vi "Register Dynamic Status Change Event.vi"() -> ()   [LabVIEW 2014]
uses:
  user.lib/_NEVSTOP/JKI State Machine ++/_Support/_JKISMQFGV.vi
  user.lib/_NEVSTOP/JKI State Machine ++/_Support/FGV-BroadcastRegistry/FGV-BroadcastRegistry.vi
  user.lib/_NEVSTOP/JKI State Machine ++/JKI-State-Machine-Plus.lvlib
panel:
  in  "unRegister":bool
  in  "Register":bool
  out "State History 2":string
  in  "Start SubModule":bool
  out "State History":string
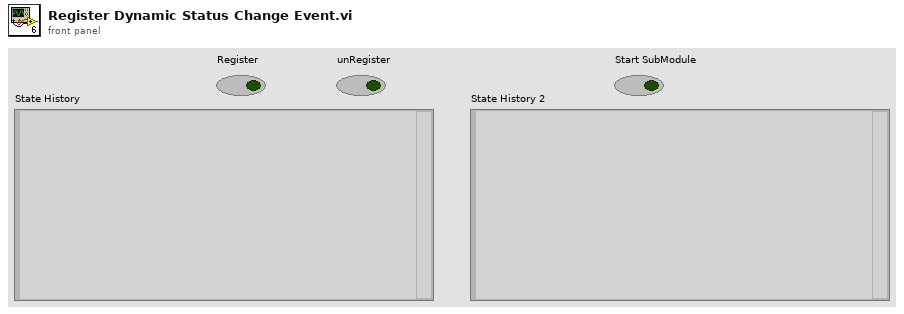
[diagram p1: front panel]
types:
  T1 = enum32{"Invalid", "Standard", "Closed", "Hidden", "Minimized", "Maximized"}
  T2 = enum32{"invalid app kind", "Development System", "Run Time System", "Student Edition", "Embedded LabVIEW", "Evaluation", "Custom"}
  T3 = cluster{"Core":cluster{"Current VI Reference":refnum<vi>, "Close Panel on Exit?":bool}, "Your Boolean data":bool, "Your string data":string}
  T4 = cluster{"Current VI Reference":refnum<vi>, "Close Panel on Exit?":bool}
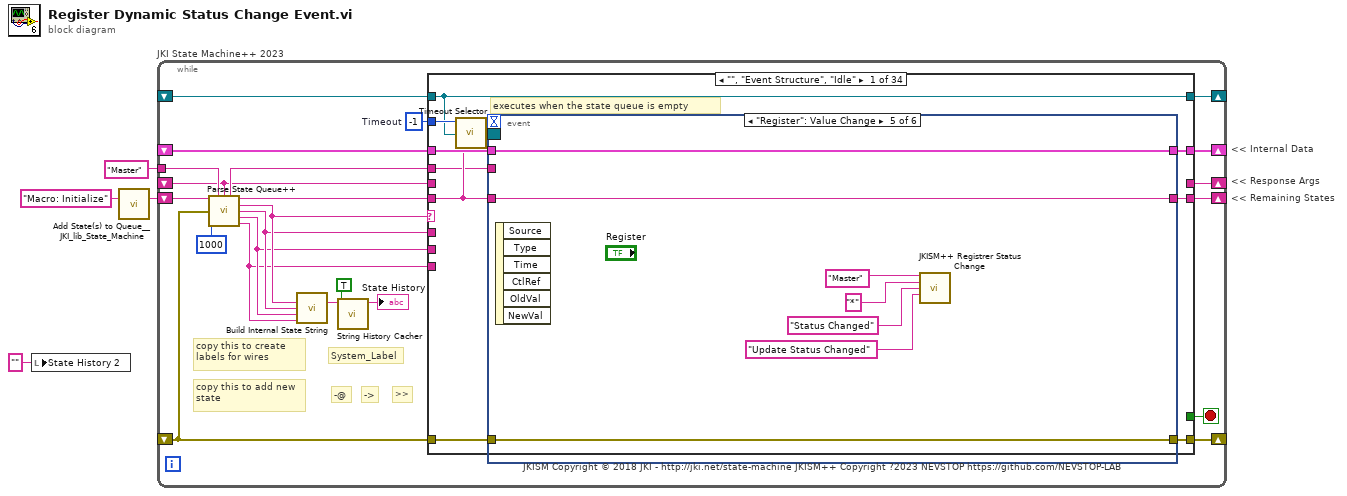
[diagram p0: block diagram]
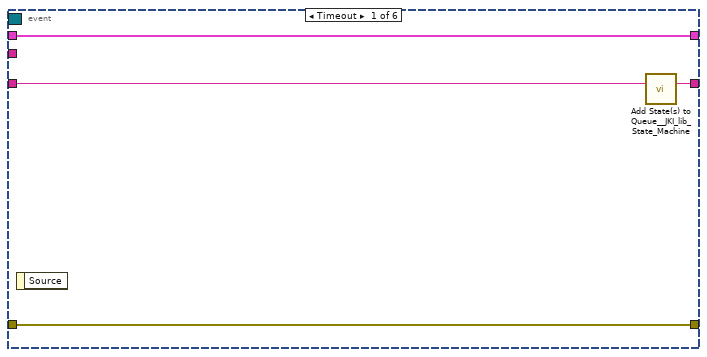
[diagram p2: hidden frame]
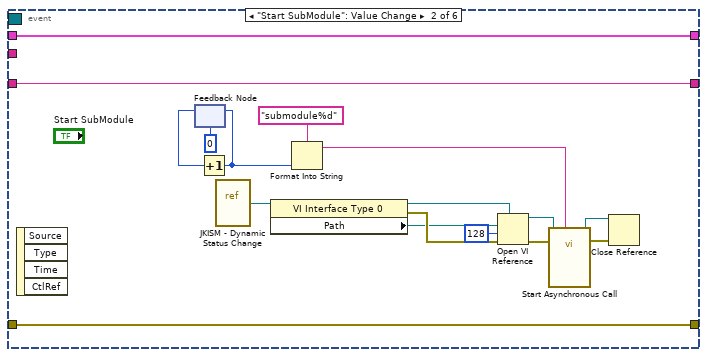
[diagram p3: hidden frame]
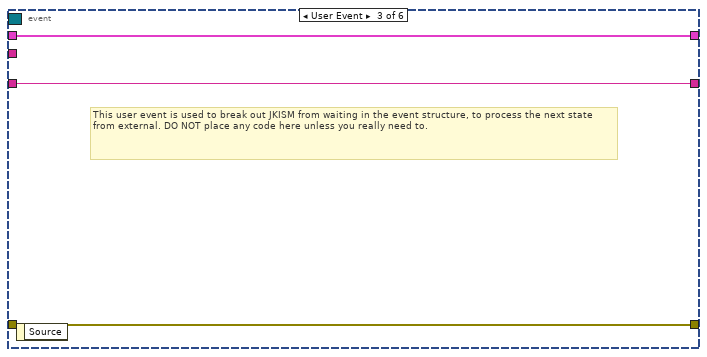
[diagram p4: hidden frame]
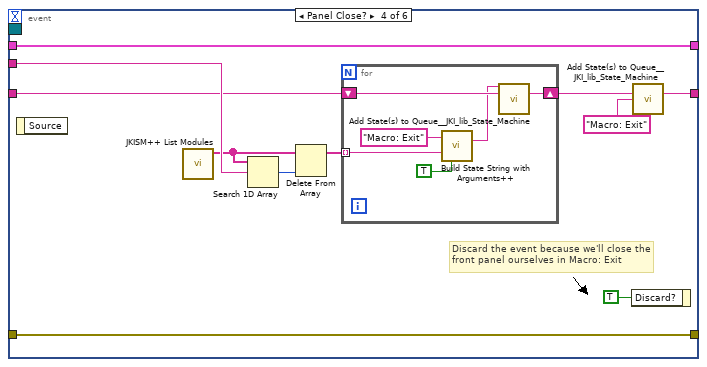
[diagram p5: hidden frame]
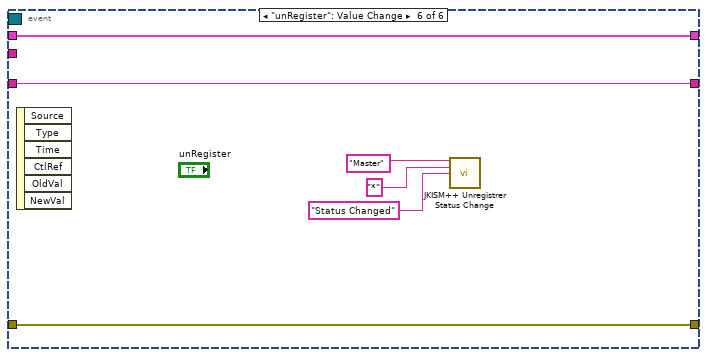
[diagram p6: hidden frame]
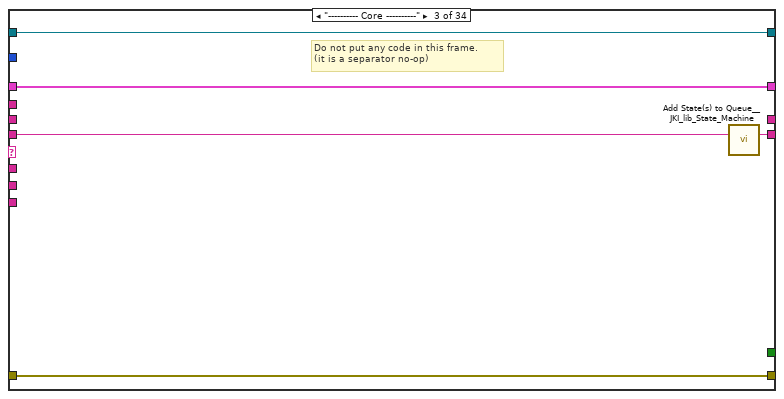
[diagram p8: hidden frame]
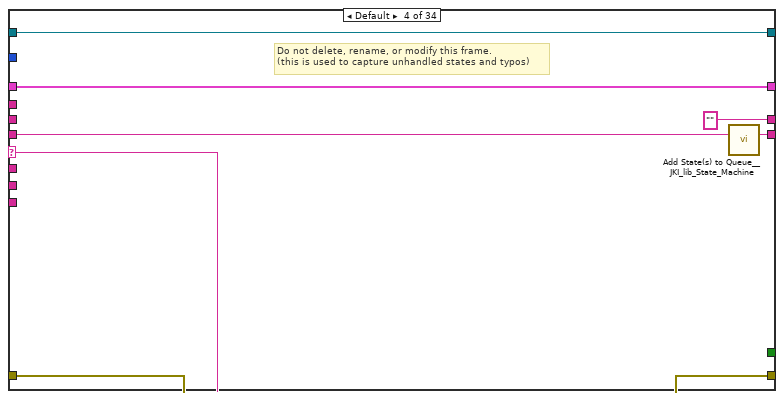
[diagram p9: hidden frame]
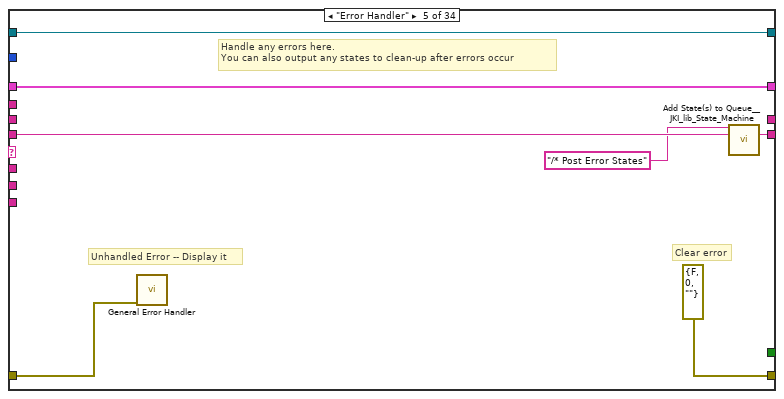
[diagram p10: hidden frame]
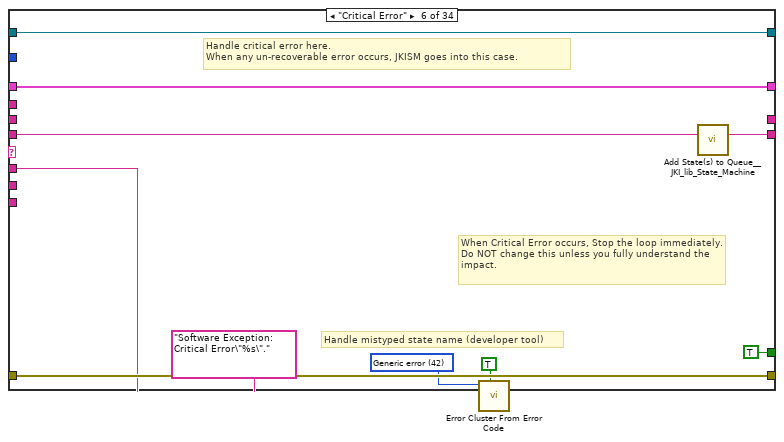
[diagram p11: hidden frame]
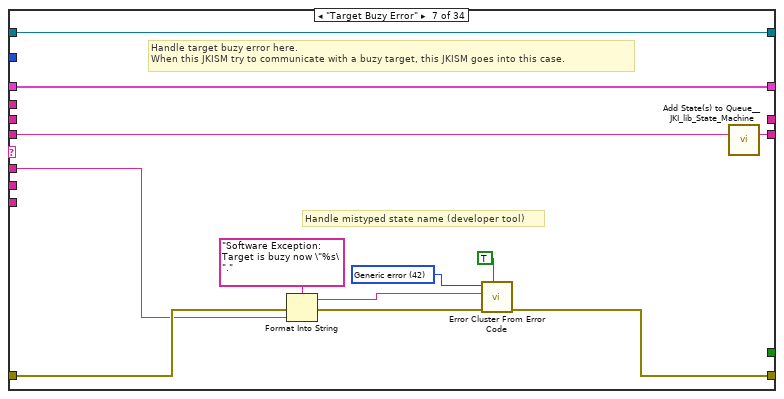
[diagram p12: hidden frame]
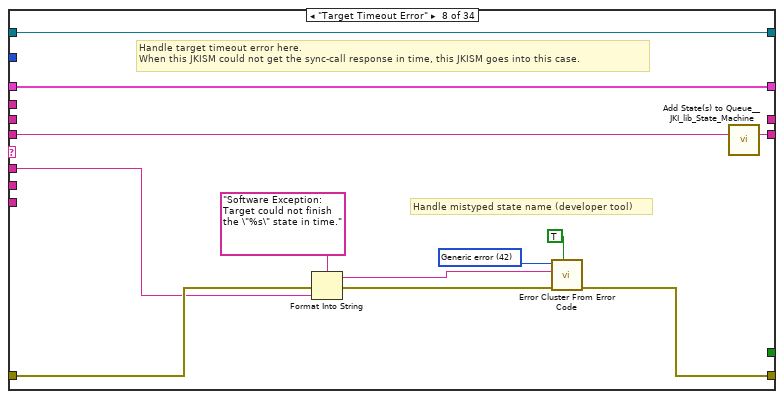
[diagram p13: hidden frame]
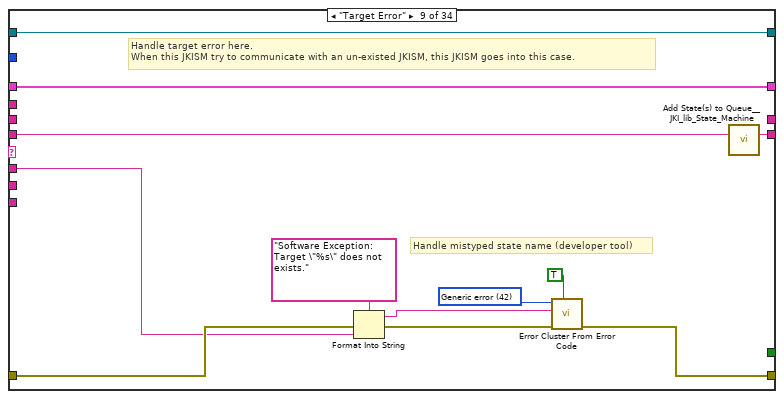
[diagram p14: hidden frame]
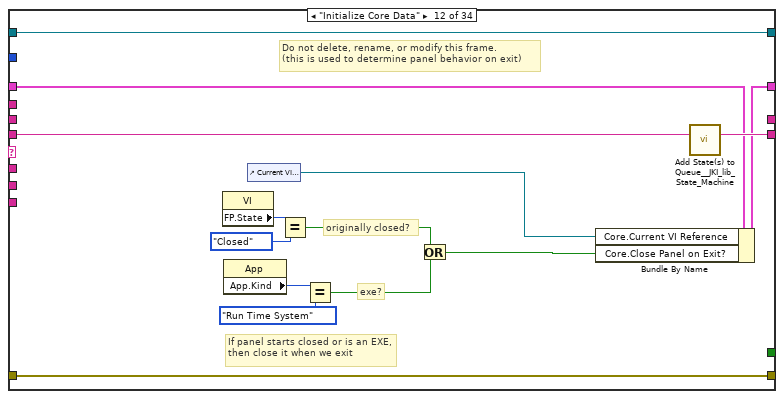
[diagram p17: hidden frame]
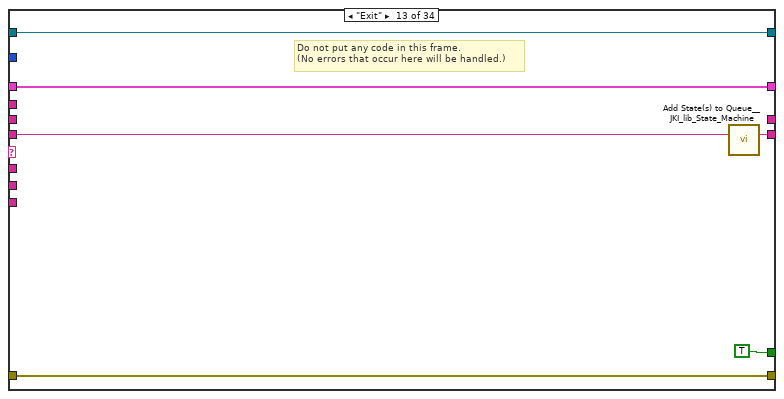
[diagram p18: hidden frame]
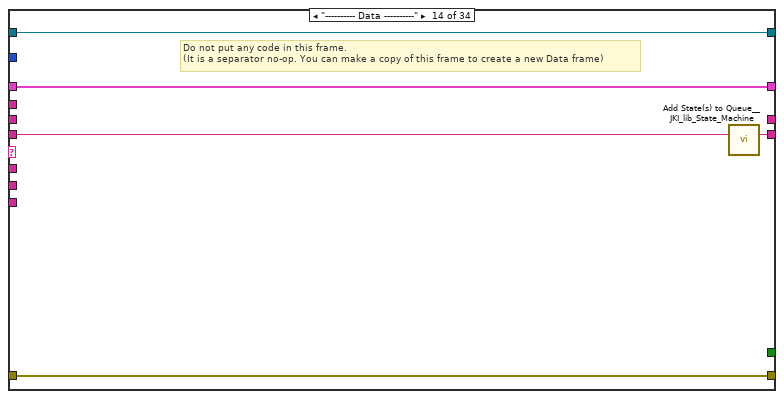
[diagram p19: hidden frame]
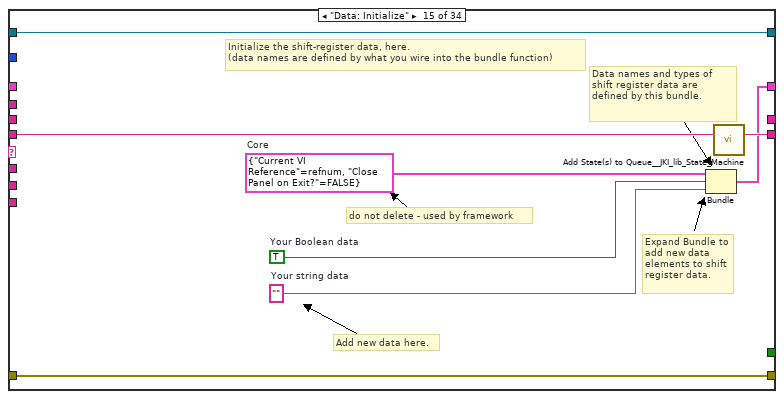
[diagram p20: hidden frame]
diagram:
  # "<< Internal Data"
  # "<< Response Args"
  # "<< Remaining States"
  n1 = local write "State History 2"("" ("State History 2")) -> ()
  n2 = call <vilib>:"Add State(s) to Queue__JKI_lib_State_Machine.vi"("State(s) in (\"\")"="Macro: Initialize") -> ("States Out"=w4:string)  [unwired: 14 in]
  n3 = while "JKI State Machine++ 2023" {
    shift-right: [w22] -> _
    shift-left: _ -> [w21]
    shift-right: [w25] -> _
    shift-left: _ -> [w19]
    shift-right: [w24] -> _
    shift-left: w4 -> [w26]
    tunnel: "Master" ("Name(\"\" to use uuid)") -> [w14]
    shift-right: [w17] -> _
    shift-left: _ -> [w6]
    shift-right: [w16] -> _
    shift-left: _ -> [w15]
    stop <- w23 stop-if-true
    w20 = -1  # Timeout
    # "JKISM Copyright © 2018 JKI - http://jki.net/state-machine JKISM++ Copyright ?2023 NEVSTOP https://github.com/NEVSTOP-LAB"
    # "copy this to add new state"
    # ">>"
    # "->"
    # "-@"
    # "copy this to create labels for wires"
    # "System_Label"
    n4 = call "Parse State Queue++.vi"("State Queue"=w26, "Name(\"\" to use uuid)"=w14, "Response Arguments"=w6, "Error In (no error)"=w19, "Response Timeout(5000ms)"=1000 ("Response Timeout(1000ms)")) -> ("Name Used"=w7:string, "Remaining States"=w27:string, "Current State"=w11:string, "Arguments"=w10:string, "Argument - State"=w9:string, "From Who"=w8:string)  [unwired: 5 in]
    n5 = call "Build Internal State String.vi"("State"=w11, "Arguments (\"\")"=w10, "Arg-State (\"\")"=w9, "Source (\"\")"=w8) -> ("State with Arguments"=w12:string)  [unwired: 11 in]
    n6 = call "String History Cacher.vi"("Include Timestamp(F)"=TRUE, "String"=w12) -> ("String Cache"=→"State History":string)  [unwired: 9 in]
    n7 = case shown="\"\", \"Event Structure\", \"Idle\"" w11 {
      selector: w11 -> [_ _ _ w103 _ _ _ _ _ _ _ _ _ _ _ _ _ _ _ _ _ _ _ _ _ _ _ _ _ _ _ _ _ _]
      tunnel: w27 -> [w29 w94 w100 w107 w120 w130 w133 w150 w162 w171 w175 w190 w196 w201 w209 w216 w221 w227 w231 w237 w242 w249 w261 w331 w337 w348 w351 w356 w362 w370 w376 w384 w391 w405]
      tunnel: w10 -> [_ _ _ _ _ w123 w135 w146 w158 _ _ _ _ _ _ _ _ _ _ _ _ w244 w255 _ _ _ _ _ w359 _ _ w378 _ w402]
      tunnel: w21 -> [w36 w93 w97 w105 w117 w131 w137 w148 w160 w170 w174 w183 w194 w198 _ w211 w218 w226 w230 w234 w240 w247 w257 w328 w334 w345 w350 w355 w361 w367 w373 w383 w388 w404]
      tunnel: [w35 w95 w98 w109 errorcluster {"status"=FALSE, "code"=0, "source"=""} ("error out") w132 w140 w152 w164 w172 w176 w187 w193 w199 w206 w212 w219 w222 w229 w235 w239 w245 w258 w329 w335 w346 w352 w357 w363 w368 w374 w385 w389 w406] -> w25
      tunnel: w19 -> [w34 w95 w98 w108 w116 w132 w139 w151 w163 w172 w176 w187 w193 w199 w206 w213 w219 _ w232 w235 w239 w246 w259 w329 w335 w346 w352 w357 w363 w368 w374 w385 w389 w406]
      tunnel: [w37 w94 w99 w106 w119 w129 w138 w149 w161 w171 w175 w189 w195 w200 w208 w215 w220 w227 w231 w236 w241 w248 w260 w330 w336 w347 w351 w356 w362 w369 w375 w384 w390 w405] -> w24
      tunnel: [_ _ _ _ _ TRUE _ _ _ _ _ _ TRUE _ _ _ _ _ _ _ _ _ _ _ _ _ _ _ _ _ _ _ _ _] -> w23
      tunnel: [w33 w93 w97 w105 w117 w131 w137 w148 w160 w170 w174 w188 w194 w198 w207 w211 w218 w226 w230 w234 w240 w247 w257 w328 w334 w345 w350 w355 w361 w367 w373 w383 w388 w404] -> w22
      tunnel: w20 -> [w32 _ _ _ _ _ _ _ _ _ _ _ _ _ _ _ _ _ _ _ _ _ _ _ _ _ _ _ _ _ _ _ _ _]
      tunnel: w8 -> [_ _ _ _ _ _ _ _ _ _ _ _ _ _ _ _ _ _ _ _ _ _ _ _ _ _ _ _ _ _ _ w379 _ w397]
      tunnel: w9 -> [_ _ _ _ _ _ _ _ _ _ _ _ _ _ _ _ _ _ _ _ _ _ _ _ _ _ _ _ _ _ _ _ _ w396]
      tunnel: [_ _ _ "" _ _ _ _ _ _ _ _ _ _ _ _ _ _ _ _ _ _ _ _ _ _ _ "API1 Response" w358 _ "DoA Finished" _ "DoB Finished" _] -> w17
      tunnel: [w31 w92 w96 w101 w114 w121 w134 w145 w157 w169 w173 w177 w191 w197 w202 w210 w217 w225 w228 w233 w238 w243 w254 w327 w332 w338 w349 w354 w360 w366 w372 w382 w387 w403] -> w16
      tunnel: w15 -> [w31 w92 w96 w101 w114 w121 w134 w145 w157 w169 w173 w177 w191 w197 w202 w210 w217 _ w228 w233 w238 w243 w254 w327 w332 w338 w349 w354 w360 w366 w372 w382 w387 w403]
      tunnel: w7 -> [w28 _ _ _ _ _ _ _ _ _ _ _ _ _ _ _ _ w224 _ _ _ _ _ _ _ _ _ _ _ _ _ _ _ _]
      tunnel: w6 -> [_ _ _ _ _ _ _ _ _ _ _ _ _ _ _ _ _ _ _ _ _ _ _ _ _ _ _ _ _ _ _ _ _ _]
      frame "", "Event Structure", "Idle" {
        # "executes when the state queue is empty"
        n8 = call "Timeout Selector.vi"("Remaining States"=w29, "Timeout Expected"=w32) -> ("Timeout"=w30:i32)  [unwired: 5 in]
        n9 = event shown="[4] \"Register\": Value Change" {
          selector: w31 -> [_ _ _ _ _ _]
          dyn-events: _ -> [_ _ _ _ _ _]
          timeout: w30 -> [_ _ _ _ _ _]
          tunnel: w29 -> [w41 w58 w60 w63 w85 w91]
          tunnel: [w40 w58 w60 w72 w85 w91] -> w37
          tunnel: w36 -> [w38 w56 w61 w70 w83 w89]
          tunnel: [w39 w57 w59 w71 w84 w90] -> w35
          tunnel: w34 -> [w39 w57 w59 w71 w84 w90]
          tunnel: [w38 w56 w61 w70 w83 w89] -> w33
          tunnel: w28 -> [_ _ _ w68 _ _]
          event Timeout {
            n10 = event-data() -> ()  [unwired: 1 in, 1 out]
            n11 = call <vilib>:"Add State(s) to Queue__JKI_lib_State_Machine.vi"("State(s) in (\"\")"=w41) -> ("States Out"=w40:string)  [unwired: 14 in]
          }
          event "Start SubModule": Value Change {
            n12 = event-data() -> ()  [unwired: 1 in, 4 out]
            n13 = feedback #1(0 ("Response Timeout(1000ms)")) -> (w54:i32)
            n14 = Increment(x=w54) -> (x+1=w44:i32)
            n15 = feedback-in #1(w44) -> ()
            n16 = vi-ref "JKISM - Dynamic Status Change.vi"() -> (w46:refnum<vi>)
            n17 = property class="VI Interface Type 0"(reference=w46) -> (reference out=w50:refnum<vi>, error out=w48:errorcluster, "Path"=w47:path)  [unwired: 1 in]
            n18 = Format Into String(format string="submodule%d", w44) -> (resulting string=w42:string)  [unwired: 2 in, 1 out]
            n19 = Open VI Reference(type specifier VI Refnum (for type only)=w50, vi path=w47, options=128, error in (no error)=w48) -> (vi reference=w49:refnum<vi>, error out=w45:errorcluster)  [unwired: 2 in]
            n20 = call-by-ref "Start Asynchronous Call"(reference=w49, error in=w45, "Name(\"\" to use uuid)"=w42) -> (reference out=w52:refnum<vi>, error out=w51:errorcluster)  [unwired: 11 in]
            n21 = Close Reference(reference=w52, error in (no error)=w51) -> ()  [unwired: 1 out]
          }
          event User Event {
            # "This user event is used to break out JKISM from waiting in the event structure, to process the next state from external. DO NOT place any code here unless you really need to."
            n22 = event-data() -> ()  [unwired: 1 in, 1 out]
          }
          event Panel Close? {
            # "Discard the event because we'll close the front panel ourselves in Macro: Exit"
            n23 = event-data() -> ()  [unwired: 1 in, 1 out]
            n24 = call "JKISM++ List Modules.vi"() -> ("Name"=w67:string[])  [unwired: 10 in, 1 out]
            n25 = Search 1D Array(1D array=w67, element=w68) -> (index of element=w66:i32)  [unwired: 1 in]
            n26 = Delete From Array(array=w67, index=w66) -> (array with subset deleted=w65:string[])  [unwired: 1 in, 1 out]
            n27 = for {
              tunnel: w65 -> [w78] mode=indexing
              shift-right: [w75] -> w64
              shift-left: w63 -> [w74]
              n28 = call "Build State String with Arguments++.vi"("State"="Macro: Exit", "Dest Module (\"\")"=w78, "Sync-Call(@) T By Default/Async-Call(->) F"=TRUE) -> ("State with Arguments"=w73:string)  [unwired: 12 in]
              n29 = call <vilib>:"Add State(s) to Queue__JKI_lib_State_Machine.vi"("State(s) in Front (\"\")"=w73, "State(s) in (\"\")"=w74) -> ("States Out"=w75:string)  [unwired: 13 in]
            }
            n30 = event-data("Discard?"=TRUE) -> ()  [unwired: 1 in, 1 out]
            n31 = call <vilib>:"Add State(s) to Queue__JKI_lib_State_Machine.vi"("State(s) in (\"\")"=w64, "State(s) at Back (\"\")"="Macro: Exit") -> ("States Out"=w72:string)  [unwired: 13 in]
          }
          event "Register": Value Change {
            n32 = event-data() -> ()  [unwired: 1 in, 6 out]
            n33 = call "JKISM++ Registrer Status Change.vi"("JKISM Name"="Master" ("Source JKISM Name"), "Source JKISM Name (* as Default)"="*" ("Name(\"\" to use uuid)"), "Status"="Status Changed" ("Message"), "ActingMsg (if \"\", same as Source Message)"="Update Status Changed" ("ActingMsg (if \"\", same as Source Message)")) -> ()  [unwired: 10 in, 2 out]
          }
          event "unRegister": Value Change {
            n34 = event-data() -> ()  [unwired: 1 in, 6 out]
            n35 = call "JKISM++ Unregistrer Status Change.vi"("JKISM Name"="Master" ("Source JKISM Name"), "Source JKISM Name"="*" ("Name(\"\" to use uuid)"), "Status"="Status Changed" ("Message")) -> ()  [unwired: 11 in, 2 out]
          }
        }
      }
      frame "JKISM++ Documentation" {
        # "JKISM++ Documentation"
        # "State Syntax:\nStateCategory: State >> Argument @|-> JKISMName\nLine Terminator: Line feed\n\nExample:\nUI: Help >> About @Main\nUI: Help >> About ->Main"
        # "Commenting:\nTo add a comment use \"//\" or \"#\" and all text to the right will be ignored\nCommenting Example:\nUI: Initialize // This initializes the UI\n# This whole line is a comment\n// Another comment line"
        # "Where \"UI\" is the state category\nWhere \"Help\" is the state\nWhere \"About\" is the argument\nWhere \"Main\" is the Name of JKISM,which actually run the \"UI: Help >> About\"\n\n    \"@\" stands for sync state. Current JKISM will wait until the state is finished. \n            - if \"Main\" named JKISM does not exist, \"Target Error\" will occur.\n            - if \"Main\" named JKISM is in another sync remote state, \"Target Buzy Error\" will occur.\n            - if \"Main\" named JKISM could not finish the state in time, \"Target Timeout Error\" will occur.\n            - if everything is right. \"Response\" will occur with Argument back from \"Main\" named JKISM. \n\n    \"->\" stands for async state. Current JKISM will post the state and continue to next state in next iteration.\n            - if \"Main\" named JKISM does not exist, \"Target Error\" will occur.\n            - if everything is right. \"Async Message Posted\" will occur.\n            - After State is finished. Caller will receive a \"Async Response\" state from callee.\n\nWhen duplicated name is used for multiple JKISM module or some framework problem happens, \"Critical Error\" will occur."
      }
      frame "---------- Core ----------" {
        # "Do not put any code in this frame.\n(it is a separator no-op)"
        n36 = call <vilib>:"Add State(s) to Queue__JKI_lib_State_Machine.vi"("State(s) in (\"\")"=w100) -> ("States Out"=w99:string)  [unwired: 14 in]
      }
      frame Default {
        w112 = 42 items=["No error", "Argument error", "Memory is full", "Out of zone", "End of file", "File already open", "Generic file I/O error", "File not found", "File permission error", "Disk is full", "Duplicate path", "Too many files open", "System feature not enabled", "Resource file not found", "Cannot add resource", "Resource not found", "Image not found", "Image memory error", "Pen does not exist", "Config type invalid", "Config token not found", "Config parse error", "Config memory error", "Bad external code format", "Bad external code offset", "External code not present", "Null window", "Destroy window error", "Null menu", "Print aborted", "Bad print record", "Print driver error", "Windows error during printing", "Memory error during printing", "Print dialog error", "Generic print error", "Invalid device refnum", "Device not found", "Device parameter error", "Device unit error", "Cannot open device", "Device call aborted", "Generic error", "Cancelled by user", "Object ID too low", "Object ID too high", "Object not in heap", "Unknown heap", "Unknown object (invalid DefProc)", "Unknown object (DefProc not in table)", "Message out of range", "Invalid (null) method", "Unknown message", "Manager call not supported", "Bad address", "Network operation in progress", "Network operation timed out", "Connection is busy", "Network attribute not supported", "Network error", "Address in use", "System out of memory", "Connection aborted", "Connection refused", "Not connected", "Already connected", "Connection closed", "Initialization error (interapplication manager)", "Bad occurrence", "Wait on unbound occurrence handler", "Occurrence queue overflow", "Datalog type conflict", "Unused", "Unrecognized type (interapplication manager)", "Memory corrupt", "Failed to make temporary DLL", "Old CIN version", "Drag socket not found", "Failed to load drop-object", "Failed to register OLE object", "Failed to release OLE object", "Format specifier type mismatch", "Unknown format specifier", "Too few format specifiers", "Too many format specifiers", "Scan failed", "Newer CIN version", "Error converting to variant", "Runtime menu error", "Password tampered", "Variant attribute not found", "Incompatible variant data type", "Event data is not available", "Event Store is not present", "Occurrence is not found", "Event Queue is not created", "Event info is not available", "Refnum passed is NULL", "Error retrieving Class GUID", "Error retrieving CoClass GUID", "Error retrieving TypeLib GUID.", "Bad built application magic bytes.", "Specific driver is different from the specific driver associated with the Logical Name.", "There is no session opened to the class driver.", "Max Error", "MAX - Error with config objects", "MAX - Error loading configuration", "MAX - Group not supported"]
        # "Do not delete, rename, or modify this frame.\n(this is used to capture unhandled states and typos)"
        # "Handle mistyped state name (developer tool)"
        n37 = Format Into String(format string="Software Exception: Unhandled State \"%s\"." ("message"), error in=w108, w103) -> (resulting string=w111:string, error out=w110:errorcluster)  [unwired: 1 in]
        n38 = call <vilib>:"Error Cluster From Error Code.vi"("show call chain? (False)"=TRUE, "error in (no error)"=w110, "error message (\"\")"=w111, "error code (0)"=w112) -> ("error out"=w109:errorcluster)  [unwired: 5 in]
        n39 = call <vilib>:"Add State(s) to Queue__JKI_lib_State_Machine.vi"("State(s) in (\"\")"=w107) -> ("States Out"=w106:string)  [unwired: 14 in]
      }
      frame "Error Handler" {
        # "Unhandled Error -- Display it"
        # "Handle any errors here.\nYou can also output any states to clean-up after errors occur"
        # "Clear error"
        n40 = call <vilib>:"General Error Handler.vi"("error in (no error)"=w116) -> ()  [unwired: 10 in, 5 out]
        n41 = call <vilib>:"Add State(s) to Queue__JKI_lib_State_Machine.vi"("State(s) in Front (\"\")"="/* Post Error States", "State(s) in (\"\")"=w120) -> ("States Out"=w119:string)  [unwired: 13 in]
      }
      frame "Critical Error" {
        w127 = 42 items=["No error", "Argument error", "Memory is full", "Out of zone", "End of file", "File already open", "Generic file I/O error", "File not found", "File permission error", "Disk is full", "Duplicate path", "Too many files open", "System feature not enabled", "Resource file not found", "Cannot add resource", "Resource not found", "Image not found", "Image memory error", "Pen does not exist", "Config type invalid", "Config token not found", "Config parse error", "Config memory error", "Bad external code format", "Bad external code offset", "External code not present", "Null window", "Destroy window error", "Null menu", "Print aborted", "Bad print record", "Print driver error", "Windows error during printing", "Memory error during printing", "Print dialog error", "Generic print error", "Invalid device refnum", "Device not found", "Device parameter error", "Device unit error", "Cannot open device", "Device call aborted", "Generic error", "Cancelled by user", "Object ID too low", "Object ID too high", "Object not in heap", "Unknown heap", "Unknown object (invalid DefProc)", "Unknown object (DefProc not in table)", "Message out of range", "Invalid (null) method", "Unknown message", "Manager call not supported", "Bad address", "Network operation in progress", "Network operation timed out", "Connection is busy", "Network attribute not supported", "Network error", "Address in use", "System out of memory", "Connection aborted", "Connection refused", "Not connected", "Already connected", "Connection closed", "Initialization error (interapplication manager)", "Bad occurrence", "Wait on unbound occurrence handler", "Occurrence queue overflow", "Datalog type conflict", "Unused", "Unrecognized type (interapplication manager)", "Memory corrupt", "Failed to make temporary DLL", "Old CIN version", "Drag socket not found", "Failed to load drop-object", "Failed to register OLE object", "Failed to release OLE object", "Format specifier type mismatch", "Unknown format specifier", "Too few format specifiers", "Too many format specifiers", "Scan failed", "Newer CIN version", "Error converting to variant", "Runtime menu error", "Password tampered", "Variant attribute not found", "Incompatible variant data type", "Event data is not available", "Event Store is not present", "Occurrence is not found", "Event Queue is not created", "Event info is not available", "Refnum passed is NULL", "Error retrieving Class GUID", "Error retrieving CoClass GUID", "Error retrieving TypeLib GUID.", "Bad built application magic bytes.", "Specific driver is different from the specific driver associated with the Logical Name.", "There is no session opened to the class driver.", "Max Error", "MAX - Error with config objects", "MAX - Error loading configuration", "MAX - Group not supported"]
        # "Handle critical error here.\nWhen any un-recoverable error occurs, JKISM goes into this case."
        # "When Critical Error occurs, Stop the loop immediately. Do NOT change this unless you fully understand the impact."
        # "Handle mistyped state name (developer tool)"
        n42 = Format Into String(format string="Software Exception: Critical Error\"%s\"." ("message"), w123) -> (resulting string=w126:string, error out=w125:errorcluster)  [unwired: 2 in]
        n43 = call <vilib>:"Error Cluster From Error Code.vi"("show call chain? (False)"=TRUE, "error in (no error)"=w125, "error message (\"\")"=w126, "error code (0)"=w127) -> ()  [unwired: 5 in, 1 out]
        n44 = call <vilib>:"Add State(s) to Queue__JKI_lib_State_Machine.vi"("State(s) in (\"\")"=w130) -> ("States Out"=w129:string)  [unwired: 14 in]
      }
      frame "Target Buzy Error" {
        w143 = 42 items=["No error", "Argument error", "Memory is full", "Out of zone", "End of file", "File already open", "Generic file I/O error", "File not found", "File permission error", "Disk is full", "Duplicate path", "Too many files open", "System feature not enabled", "Resource file not found", "Cannot add resource", "Resource not found", "Image not found", "Image memory error", "Pen does not exist", "Config type invalid", "Config token not found", "Config parse error", "Config memory error", "Bad external code format", "Bad external code offset", "External code not present", "Null window", "Destroy window error", "Null menu", "Print aborted", "Bad print record", "Print driver error", "Windows error during printing", "Memory error during printing", "Print dialog error", "Generic print error", "Invalid device refnum", "Device not found", "Device parameter error", "Device unit error", "Cannot open device", "Device call aborted", "Generic error", "Cancelled by user", "Object ID too low", "Object ID too high", "Object not in heap", "Unknown heap", "Unknown object (invalid DefProc)", "Unknown object (DefProc not in table)", "Message out of range", "Invalid (null) method", "Unknown message", "Manager call not supported", "Bad address", "Network operation in progress", "Network operation timed out", "Connection is busy", "Network attribute not supported", "Network error", "Address in use", "System out of memory", "Connection aborted", "Connection refused", "Not connected", "Already connected", "Connection closed", "Initialization error (interapplication manager)", "Bad occurrence", "Wait on unbound occurrence handler", "Occurrence queue overflow", "Datalog type conflict", "Unused", "Unrecognized type (interapplication manager)", "Memory corrupt", "Failed to make temporary DLL", "Old CIN version", "Drag socket not found", "Failed to load drop-object", "Failed to register OLE object", "Failed to release OLE object", "Format specifier type mismatch", "Unknown format specifier", "Too few format specifiers", "Too many format specifiers", "Scan failed", "Newer CIN version", "Error converting to variant", "Runtime menu error", "Password tampered", "Variant attribute not found", "Incompatible variant data type", "Event data is not available", "Event Store is not present", "Occurrence is not found", "Event Queue is not created", "Event info is not available", "Refnum passed is NULL", "Error retrieving Class GUID", "Error retrieving CoClass GUID", "Error retrieving TypeLib GUID.", "Bad built application magic bytes.", "Specific driver is different from the specific driver associated with the Logical Name.", "There is no session opened to the class driver.", "Max Error", "MAX - Error with config objects", "MAX - Error loading configuration", "MAX - Group not supported"]
        # "Handle target buzy error here.\nWhen this JKISM try to communicate with a buzy target, this JKISM goes into this case."
        # "Handle mistyped state name (developer tool)"
        n45 = Format Into String(format string="Software Exception: Target is buzy now \"%s\"." ("message"), error in=w139, w135) -> (resulting string=w142:string, error out=w141:errorcluster)  [unwired: 1 in]
        n46 = call <vilib>:"Error Cluster From Error Code.vi"("show call chain? (False)"=TRUE, "error in (no error)"=w141, "error message (\"\")"=w142, "error code (0)"=w143) -> ("error out"=w140:errorcluster)  [unwired: 5 in]
        n47 = call <vilib>:"Add State(s) to Queue__JKI_lib_State_Machine.vi"("State(s) in (\"\")"=w133) -> ("States Out"=w138:string)  [unwired: 14 in]
      }
      frame "Target Timeout Error" {
        w155 = 42 items=["No error", "Argument error", "Memory is full", "Out of zone", "End of file", "File already open", "Generic file I/O error", "File not found", "File permission error", "Disk is full", "Duplicate path", "Too many files open", "System feature not enabled", "Resource file not found", "Cannot add resource", "Resource not found", "Image not found", "Image memory error", "Pen does not exist", "Config type invalid", "Config token not found", "Config parse error", "Config memory error", "Bad external code format", "Bad external code offset", "External code not present", "Null window", "Destroy window error", "Null menu", "Print aborted", "Bad print record", "Print driver error", "Windows error during printing", "Memory error during printing", "Print dialog error", "Generic print error", "Invalid device refnum", "Device not found", "Device parameter error", "Device unit error", "Cannot open device", "Device call aborted", "Generic error", "Cancelled by user", "Object ID too low", "Object ID too high", "Object not in heap", "Unknown heap", "Unknown object (invalid DefProc)", "Unknown object (DefProc not in table)", "Message out of range", "Invalid (null) method", "Unknown message", "Manager call not supported", "Bad address", "Network operation in progress", "Network operation timed out", "Connection is busy", "Network attribute not supported", "Network error", "Address in use", "System out of memory", "Connection aborted", "Connection refused", "Not connected", "Already connected", "Connection closed", "Initialization error (interapplication manager)", "Bad occurrence", "Wait on unbound occurrence handler", "Occurrence queue overflow", "Datalog type conflict", "Unused", "Unrecognized type (interapplication manager)", "Memory corrupt", "Failed to make temporary DLL", "Old CIN version", "Drag socket not found", "Failed to load drop-object", "Failed to register OLE object", "Failed to release OLE object", "Format specifier type mismatch", "Unknown format specifier", "Too few format specifiers", "Too many format specifiers", "Scan failed", "Newer CIN version", "Error converting to variant", "Runtime menu error", "Password tampered", "Variant attribute not found", "Incompatible variant data type", "Event data is not available", "Event Store is not present", "Occurrence is not found", "Event Queue is not created", "Event info is not available", "Refnum passed is NULL", "Error retrieving Class GUID", "Error retrieving CoClass GUID", "Error retrieving TypeLib GUID.", "Bad built application magic bytes.", "Specific driver is different from the specific driver associated with the Logical Name.", "There is no session opened to the class driver.", "Max Error", "MAX - Error with config objects", "MAX - Error loading configuration", "MAX - Group not supported"]
        # "Handle target timeout error here.\nWhen this JKISM could not get the sync-call response in time, this JKISM goes into this case."
        # "Handle mistyped state name (developer tool)"
        n48 = Format Into String(format string="Software Exception: Target could not finish the \"%s\" state in time." ("message"), error in=w151, w146) -> (resulting string=w154:string, error out=w153:errorcluster)  [unwired: 1 in]
        n49 = call <vilib>:"Error Cluster From Error Code.vi"("show call chain? (False)"=TRUE, "error in (no error)"=w153, "error message (\"\")"=w154, "error code (0)"=w155) -> ("error out"=w152:errorcluster)  [unwired: 5 in]
        n50 = call <vilib>:"Add State(s) to Queue__JKI_lib_State_Machine.vi"("State(s) in (\"\")"=w150) -> ("States Out"=w149:string)  [unwired: 14 in]
      }
      frame "Target Error" {
        w167 = 42 items=["No error", "Argument error", "Memory is full", "Out of zone", "End of file", "File already open", "Generic file I/O error", "File not found", "File permission error", "Disk is full", "Duplicate path", "Too many files open", "System feature not enabled", "Resource file not found", "Cannot add resource", "Resource not found", "Image not found", "Image memory error", "Pen does not exist", "Config type invalid", "Config token not found", "Config parse error", "Config memory error", "Bad external code format", "Bad external code offset", "External code not present", "Null window", "Destroy window error", "Null menu", "Print aborted", "Bad print record", "Print driver error", "Windows error during printing", "Memory error during printing", "Print dialog error", "Generic print error", "Invalid device refnum", "Device not found", "Device parameter error", "Device unit error", "Cannot open device", "Device call aborted", "Generic error", "Cancelled by user", "Object ID too low", "Object ID too high", "Object not in heap", "Unknown heap", "Unknown object (invalid DefProc)", "Unknown object (DefProc not in table)", "Message out of range", "Invalid (null) method", "Unknown message", "Manager call not supported", "Bad address", "Network operation in progress", "Network operation timed out", "Connection is busy", "Network attribute not supported", "Network error", "Address in use", "System out of memory", "Connection aborted", "Connection refused", "Not connected", "Already connected", "Connection closed", "Initialization error (interapplication manager)", "Bad occurrence", "Wait on unbound occurrence handler", "Occurrence queue overflow", "Datalog type conflict", "Unused", "Unrecognized type (interapplication manager)", "Memory corrupt", "Failed to make temporary DLL", "Old CIN version", "Drag socket not found", "Failed to load drop-object", "Failed to register OLE object", "Failed to release OLE object", "Format specifier type mismatch", "Unknown format specifier", "Too few format specifiers", "Too many format specifiers", "Scan failed", "Newer CIN version", "Error converting to variant", "Runtime menu error", "Password tampered", "Variant attribute not found", "Incompatible variant data type", "Event data is not available", "Event Store is not present", "Occurrence is not found", "Event Queue is not created", "Event info is not available", "Refnum passed is NULL", "Error retrieving Class GUID", "Error retrieving CoClass GUID", "Error retrieving TypeLib GUID.", "Bad built application magic bytes.", "Specific driver is different from the specific driver associated with the Logical Name.", "There is no session opened to the class driver.", "Max Error", "MAX - Error with config objects", "MAX - Error loading configuration", "MAX - Group not supported"]
        # "Handle target error here.\nWhen this JKISM try to communicate with an un-existed JKISM, this JKISM goes into this case."
        # "Handle mistyped state name (developer tool)"
        n51 = Format Into String(format string="Software Exception: Target \"%s\" does not exists." ("message"), error in=w163, w158) -> (resulting string=w166:string, error out=w165:errorcluster)  [unwired: 1 in]
        n52 = call <vilib>:"Error Cluster From Error Code.vi"("show call chain? (False)"=TRUE, "error in (no error)"=w165, "error message (\"\")"=w166, "error code (0)"=w167) -> ("error out"=w164:errorcluster)  [unwired: 5 in]
        n53 = call <vilib>:"Add State(s) to Queue__JKI_lib_State_Machine.vi"("State(s) in (\"\")"=w162) -> ("States Out"=w161:string)  [unwired: 14 in]
      }
      frame "Async Response", "Response" {
        # "Handle Async-call Response (\"Async Response\" for ->)"
        # "Handle Sync-call Response (\"Response\" for @)"
        # "After Message is excuted, JKISM+ goes to this state for recieve the response. \n    For Async Message(->), \"Async Response\" is used. This JKISM will goes to \"Async Message Posted\" immediately and recieve the \"Async Response\" after the callee finishes the message.\n    For Sync Message(@),  This JKISM will wait until the message is done and immidieatly goes to \"Response\""
      }
      frame "Async Message Posted" {
        # "Handle post action for async message (->)."
        # "After Async Message is posted (->), JKISM+ goes to this state for post-action. You can use Argument - State to tell which Async Message is called."
      }
      frame "Initialize Core Data" {
        # "Do not delete, rename, or modify this frame.\n(this is used to determine panel behavior on exit)"
        # "originally closed?"
        # "exe?"
        # "If panel starts closed or is an EXE, then close it when we exit"
        n54 = property class="VI"() -> ("FP.State"=w180:T1)  [unwired: 2 in, 2 out]
        n55 = property class="App"() -> ("App.Kind"=w186:T2)  [unwired: 2 in, 2 out]
        n56 = control-ref of="Current VI Reference"() -> (w181:refnum<vi>)
        n57 = Equal?(x=w180, y=T1."Closed" ("Front Panel Window:State")) -> (x = y?=w178:bool)
        n58 = Equal?(x=w186, y=T2."Run Time System" ("Application:Kind")) -> (x = y?=w184:bool)
        n59 = Or(x=w178, y=w184) -> (x .or. y?=w182:bool)
        n60 = Bundle By Name(cluster=w183, "Core.Current VI Reference"=w181, "Core.Close Panel on Exit?"=w182) -> (w188:T3)
        n61 = call <vilib>:"Add State(s) to Queue__JKI_lib_State_Machine.vi"("State(s) in (\"\")"=w190) -> ("States Out"=w189:string)  [unwired: 14 in]
      }
      frame "Exit" {
        # "Do not put any code in this frame.\n(No errors that occur here will be handled.)"
        n62 = call <vilib>:"Add State(s) to Queue__JKI_lib_State_Machine.vi"("State(s) in (\"\")"=w196) -> ("States Out"=w195:string)  [unwired: 14 in]
      }
      frame "---------- Data ----------" {
        # "Do not put any code in this frame.\n(It is a separator no-op. You can make a copy of this frame to create a new Data frame)"
        n63 = call <vilib>:"Add State(s) to Queue__JKI_lib_State_Machine.vi"("State(s) in (\"\")"=w201) -> ("States Out"=w200:string)  [unwired: 14 in]
      }
      frame "Data: Initialize" {
        w203 = T4 {"Current VI Reference"=refnum, "Close Panel on Exit?"=FALSE}  # Core
        w205 = TRUE  # Your Boolean data
        w204 = ""  # Your string data
        # "do not delete - used by framework"
        # "Expand Bundle to add new data elements to shift register data."
        # "Add new data here."
        # "Data names and types of shift register data are defined by this bundle."
        # "Initialize the shift-register data, here.\n(data names are defined by what you wire into the bundle function)"
        n64 = Bundle("Core"=w203, "Your Boolean data"=w205, "Your string data"=w204) -> (w207:T3)  [unwired: 1 in]
        n65 = call <vilib>:"Add State(s) to Queue__JKI_lib_State_Machine.vi"("State(s) in (\"\")"=w209) -> ("States Out"=w208:string)  [unwired: 14 in]
      }
      frame "Data: Cleanup" {
        # "Cleanup any data and references, here.\n(this is called automatically, by the Macro: Exit)"
        n66 = Unbundle By Name(w211) -> ("Core.Current VI Reference"=w214:refnum<vi>)
        n67 = Close Reference(reference=w214, error in (no error)=w213) -> (error out=w212:errorcluster)
        n68 = call <vilib>:"Add State(s) to Queue__JKI_lib_State_Machine.vi"("State(s) in (\"\")"=w216) -> ("States Out"=w215:string)  [unwired: 14 in]
      }
      frame "---------- Events ----------" {
        # "Do not put any code in this frame.\n(It is a separator no-op. You can make a copy of this frame to create a new UI frame)"
        n69 = call <vilib>:"Add State(s) to Queue__JKI_lib_State_Machine.vi"("State(s) in (\"\")"=w221) -> ("States Out"=w220:string)  [unwired: 14 in]
      }
      frame "Events: Register" {
        # "Register message event to break Waiting in Event structure."
        n70 = call "JKISM++ Get New State Notifier Event.vi"("Name(\"\" to use uuid) in"=w224) -> ("Error out"=w222:errorcluster, "New State Notifier Event"=w223:refnum<user-event>)  [unwired: 9 in]
        n71 = register-events(w223) -> (reference out=w225:refnum<event-registration>)  [unwired: 2 in, 1 out]
      }
      frame "Events: Unregister" {
        n72 = Unregister For Events(event registration refnum=w228, error in=w232) -> (error out=w229:errorcluster)
      }
      frame "---------- UI ----------" {
        # "Do not put any code in this frame.\n(It is a separator no-op. You can make a copy of this frame to create a new UI frame)"
        n73 = call <vilib>:"Add State(s) to Queue__JKI_lib_State_Machine.vi"("State(s) in (\"\")"=w237) -> ("States Out"=w236:string)  [unwired: 14 in]
      }
      frame "UI: Initialize" {
        # "Initialize the User Interface, here.\n(this is called automatically, by the Macro: Init)"
        n74 = call <vilib>:"Add State(s) to Queue__JKI_lib_State_Machine.vi"("State(s) in (\"\")"=w242) -> ("States Out"=w241:string)  [unwired: 14 in]
      }
      frame "UI: Cursor Set" {
        # "Argument"
        # "Set and Unset Cursor Busy.\n(Usage: \"UI: Cursor Set >> Busy|Idle\")"
        n75 = case shown="\"Idle\", Default" w244 {
          tunnel: w246 -> [w251 w253]
          tunnel: [w250 w252] -> w245
          frame "Idle", Default {
            n76 = call <vilib>:"Unset Busy.vi"("error in (no error)"=w251) -> ("error out"=w250:errorcluster)  [unwired: 10 in]
          }
          frame "Busy" {
            n77 = call <vilib>:"Set Busy.vi"("error in (no error)"=w253) -> ("error out"=w252:errorcluster)  [unwired: 9 in, 1 out]
          }
        }
        n78 = call <vilib>:"Add State(s) to Queue__JKI_lib_State_Machine.vi"("State(s) in (\"\")"=w249) -> ("States Out"=w248:string)  [unwired: 14 in]
      }
      frame "UI: Front Panel State" {
        # "Argument"
        # "Set Front Panel Open or Closed\n(Usage: \"UI: Front Panel State >> Open|Close\")"
        n79 = Unbundle By Name(w257) -> ("Core.Current VI Reference"=w256:refnum<vi>)
        n80 = case shown="\"Minimize\", \"Minimized\"" w255 {
          tunnel: w259 -> [w267 w282 w293 w306 w319]
          tunnel: [w269 w283 w295 w308 w321] -> w258
          tunnel: w256 -> [w268 w280 w294 w307 w320]
          frame "Open", "Standard", Default {
            w262 = T1."Standard" ("State")
            n81 = property class="VI"(reference=w268, error in=w267) -> (reference out=w265:refnum<vi>, error out=w266:errorcluster, "FP.State"=w264:T1)
            n82 = Not Equal?(x=w264, y=w262) -> (x != y?=w263:bool)
            n83 = case shown="True" w263 {
              tunnel: [w273 w275] -> w269
              tunnel: w266 -> [w272 w275]
              tunnel: w265 -> [w271 _]
              tunnel: w262 -> [w270 _]
              frame True {
                n84 = invoke class="VI" method="FP.Open"(reference=w271, error in=w272, "Activate"=TRUE, "State"=w270) -> (error out=w273:errorcluster)  [unwired: 1 in, 4 out]
              }
              frame False {
              }
            }
          }
          frame "Close", "Closed" {
            n85 = property class="VI"(reference=w280, error in=w282) -> (reference out=w279:refnum<vi>, error out=w281:errorcluster, "FP.State"=w277:T1)
            n86 = Not Equal?(x=w277, y=T1."Closed" ("Front Panel Window:State")) -> (x != y?=w276:bool)
            n87 = case shown="True" w276 {
              tunnel: [w284 w287] -> w283
              tunnel: w281 -> [w284 w286]
              tunnel: w279 -> [_ w285]
              frame False {
              }
              frame True {
                n88 = invoke class="VI" method="FP.Close"(reference=w285, error in=w286) -> (error out=w287:errorcluster)  [unwired: 1 in, 2 out]
              }
            }
          }
          frame "Hidden", "Hide" {
            w288 = T1."Hidden" ("State")
            n89 = property class="VI"(reference=w294, error in=w293) -> (reference out=w291:refnum<vi>, error out=w292:errorcluster, "FP.State"=w290:T1)
            n90 = Not Equal?(x=w290, y=w288) -> (x != y?=w289:bool)
            n91 = case shown="True" w289 {
              tunnel: [w299 w300] -> w295
              tunnel: w292 -> [w298 w300]
              tunnel: w291 -> [w297 _]
              tunnel: w288 -> [w296 _]
              frame True {
                n92 = invoke class="VI" method="FP.Open"(reference=w297, error in=w298, "State"=w296) -> (error out=w299:errorcluster)  [unwired: 2 in, 4 out]
              }
              frame False {
              }
            }
          }
          frame "Minimize", "Minimized" {
            w301 = T1."Minimized" ("State")
            n93 = property class="VI"(reference=w307, error in=w306) -> (reference out=w304:refnum<vi>, error out=w305:errorcluster, "FP.State"=w303:T1)
            n94 = Not Equal?(x=w303, y=w301) -> (x != y?=w302:bool)
            n95 = case shown="True" w302 {
              tunnel: [w312 w313] -> w308
              tunnel: w305 -> [w311 w313]
              tunnel: w304 -> [w310 _]
              tunnel: w301 -> [w309 _]
              frame True {
                n96 = invoke class="VI" method="FP.Open"(reference=w310, error in=w311, "State"=w309) -> (error out=w312:errorcluster)  [unwired: 2 in, 4 out]
              }
              frame False {
              }
            }
          }
          frame "Maximize", "Maximized" {
            w314 = T1."Maximized" ("State")
            n97 = property class="VI"(reference=w320, error in=w319) -> (reference out=w317:refnum<vi>, error out=w318:errorcluster, "FP.State"=w316:T1)
            n98 = Not Equal?(x=w316, y=w314) -> (x != y?=w315:bool)
            n99 = case shown="True" w315 {
              tunnel: [w325 w326] -> w321
              tunnel: w318 -> [w324 w326]
              tunnel: w317 -> [w323 _]
              tunnel: w314 -> [w322 _]
              frame True {
                n100 = invoke class="VI" method="FP.Open"(reference=w323, error in=w324, "State"=w322) -> (error out=w325:errorcluster)  [unwired: 2 in, 4 out]
              }
              frame False {
              }
            }
          }
        }
        n101 = call <vilib>:"Add State(s) to Queue__JKI_lib_State_Machine.vi"("State(s) in (\"\")"=w261) -> ("States Out"=w260:string)  [unwired: 14 in]
      }
      frame "---------- Macro ----------" {
        # "Do not put any code in this frame.\n(It is a separator no-op. You can make a copy of this frame to create a new Macro frame)"
        n102 = call <vilib>:"Add State(s) to Queue__JKI_lib_State_Machine.vi"("State(s) in (\"\")"=w331) -> ("States Out"=w330:string)  [unwired: 14 in]
      }
      frame "Macro: Initialize" {
        w333 = "Data: Initialize\nInitialize Core Data\nEvents: Register\nUI: Initialize\nUI: Front Panel State >> Open"  # Data: Initialize Initialize Core Data Events: Register UI: Initialize UI: Front Panel State >> Open
        # "Initialization Macro\n(This is called once, when the VI starts)"
        n103 = call <vilib>:"Add State(s) to Queue__JKI_lib_State_Machine.vi"("State(s) in Front (\"\")"=w333, "State(s) in (\"\")"=w337) -> ("States Out"=w336:string)  [unwired: 13 in]
      }
      frame "Macro: Exit" {
        # "Exit Macro\n(This is called once, when the VI exits)"
        n104 = Unbundle By Name(w345) -> ("Core.Close Panel on Exit?"=w344:bool)
        n105 = Select(t="UI: Front Panel State >> Close", s=w344, f="") -> (s? t:f=w341:string)
        n106 = call <vilib>:"Add State(s) to Queue__JKI_lib_State_Machine.vi"("State(s) in (\"\")"=w341, "State(s) at Back (\"\")"="Data: Cleanup\nEvents: Unregister\nExit") -> ("States Out"=w339:string)  [unwired: 13 in]
        n107 = call <vilib>:"Add State(s) to Queue__JKI_lib_State_Machine.vi"("State(s) in Front (\"\")"=w339, "State(s) in (\"\")"=w348) -> ("States Out"=w347:string)  [unwired: 13 in]
      }
      frame "---------- API ----------" {
        # "Do not put any code in this frame.\n(It is a separator no-op. This category is recommanded to use for external API)"
      }
      frame "API: API1" {
        # "If you need to tell who triggered this state , use this string. If it's this case itself, this string is \"\"."
        # "Deal with the parameter if any"
        # "Connect this to return the response of your API"
        # "Copy/Rename this case for your own API"
      }
      frame "API: API2" {
        # "unpack HexStr  to Variant\nif complex parameter is needed."
        # "Copy/Rename this case for your own API"
        n108 = call "JKISM++ Convert HexStr to Data.vi"("HEX String"=w359) -> ()  [unwired: 8 in, 1 out]
        n109 = disable-structure shown="Enabled" {
          disable-tunnel: [w364 "API2 Response"] -> w358
          frame Disabled {
            # "pack variant to hexstr \nif complex response is needed."
            # "complex Response"
            n110 = call "JKISM++ Convert Data to HexStr.vi"() -> ("HEX String (0-9,A-F)"=w364:string)  [unwired: 9 in]
          }
          frame Enabled {
          }
        }
      }
      frame "---------- DoSth ----------" {
        # "Template Separator\n(You can make a copy of, or modify, this frame)"
        n111 = call <vilib>:"Add State(s) to Queue__JKI_lib_State_Machine.vi"("State(s) in (\"\")"=w370) -> ("States Out"=w369:string)  [unwired: 14 in]
      }
      frame "DoSth: DoA" {
        # "Your code here.\n(You can make a copy of, or modify, this frame)"
        n112 = call <vilib>:"Add State(s) to Queue__JKI_lib_State_Machine.vi"("State(s) in (\"\")"=w376) -> ("States Out"=w375:string)  [unwired: 14 in]
      }
      frame "Update Status Changed" {
        n113 = Format Into String(w379, w378) -> (resulting string=w377:string)  [unwired: 3 in, 1 out]
        n114 = call "String History Cacher.vi"("Include Timestamp(F)"=TRUE, "String"=w377) -> ("String Cache"=→"State History 2":string)  [unwired: 9 in]
      }
      frame "DoSth: DoB" {
        # "Your code here.\n(You can make a copy of, or modify, this frame)"
        n115 = call <vilib>:"Add State(s) to Queue__JKI_lib_State_Machine.vi"("State(s) in (\"\")"=w391) -> ("States Out"=w390:string)  [unwired: 14 in]
      }
      frame "Handler: Error Occured" {
        n116 = call "JKISM++ Convert HexStr to Data.vi"("HEX String"=w402) -> ("Variant"=w401:variant)  [unwired: 8 in]
        n117 = Variant To Data(type=errorcluster {"status"=FALSE, "code"=0, "source"=""} ("error in (no error)"), Variant=w401) -> (data=w399:errorcluster)  [unwired: 1 in, 1 out]
        n118 = Unbundle By Name(w399) -> ("source"=w398:string)
        n119 = Concatenate Strings("From:" ("string"), w397) -> (w395:string)
        n120 = Concatenate Strings("Because:" ("string"), w396) -> (w394:string)
        n121 = Two Button Dialog(message=w398, 1:w394, 2:w395) -> ()  [unwired: 1 out]
      }
    }
  }
